vi "test - GB2312.vi"(8 "error in (no error)":errorcluster, 11 "TestCase in":refnum<class "labview-config-library.lvclass">) -> (0 "error out":errorcluster, 3 "TestCase out":refnum<class "labview-config-library.lvclass">)   [LabVIEW 2017, in "labview-config-library.lvclass"]
uses:
  labview-config-library.lvclass
  <vilib>/addons/_JKI Toolkits/VI Tester/TestCase.llb/TestCase.lvclass
  INI-Static-Variable-Support/LabVIEW-Config/LabVIEW-Config.lvclass
  INI-Static-Variable-Support/LabVIEW-Config/Read Key (String).vi
  C:/Program Files (x86)/National Instruments/LabVIEW 2017/vi.lib/addons/_JKI Toolkits/VI Tester/TestCase.llb/TestCase.lvclass
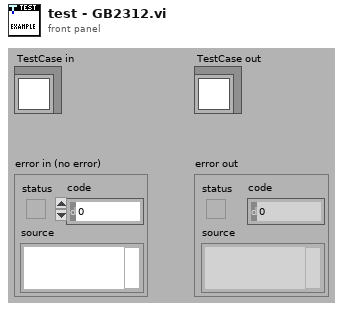
[diagram p1: front panel]
types:
  T1 = typedef "LabVIEW-Config.lvlib/LabVIEW-Config.lvclass/Config.ctl" = cluster{"Path":path, "Lines":string[], "Tokens":T2[], "Modified?":bool, "Cache":cluster{"Valid?":bool, "Key Information":T3[]}}
  T2 = typedef "LabVIEW-Config.lvlib/LabVIEW-Config.lvclass/LineToken.ctl" = enum8{"comment", "section", "key", "more"}
  T3 = typedef "LabVIEW-Config.lvlib/LabVIEW-Config.lvclass/KeyInfo.ctl" = cluster{"Key Indexes":cluster{"Indexes":i32[]}[], "Session Found?":bool, "Key found?":bool, "Session Index":i32}
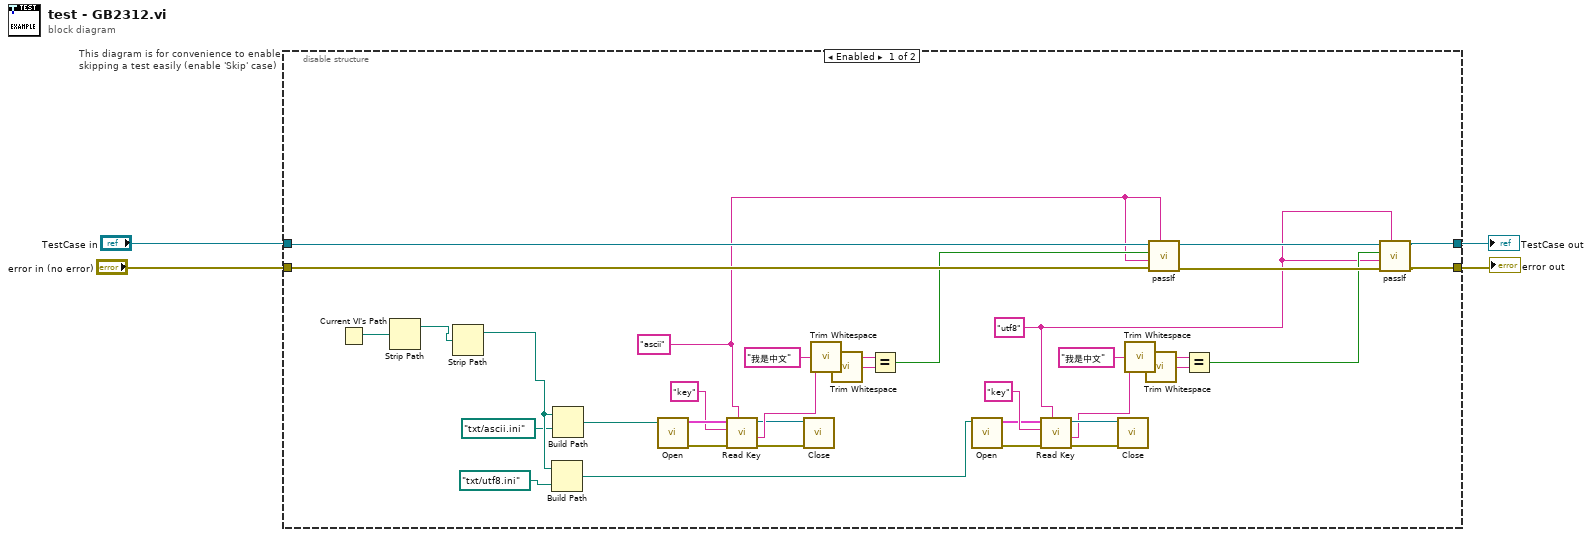
[diagram p0: block diagram]
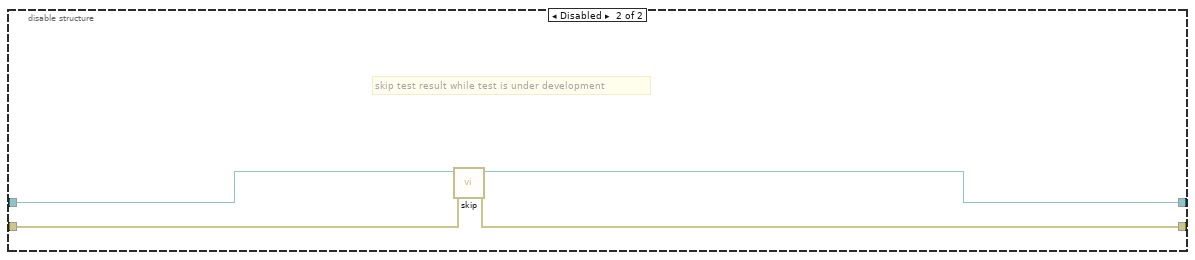
[diagram p2: hidden frame]
diagram:
  n1 = disable-structure "This diagram is for convenience to enable skipping a test easily (enable 'Skip' case)" shown="Enabled" {
    disable-tunnel: "TestCase in" -> [w12 w43]
    disable-tunnel: [w39 w41] -> w1
    disable-tunnel: [w38 w42] -> w3
    disable-tunnel: "error in (no error)" -> [w11 w40]
    frame Enabled {
      w5 = "utf8" ("Section Name")
      w7 = "ascii" ("Section Name")
      n2 = Current VI's Path() -> (path=w27:path)
      n3 = Strip Path(path=w27) -> (stripped path=w28:path)  [unwired: 1 out]
      n4 = Strip Path(path=w28) -> (stripped path=w29:path)  [unwired: 1 out]
      n5 = Build Path(base path=w29, name or relative path=path "txt/utf8.ini" ("file path (use dialog)")) -> (appended path=w13:path)
      n6 = Build Path(base path=w29, name or relative path=path "txt/ascii.ini" ("file path (use dialog)")) -> (appended path=w34:path)
      n7 = call "Open.vi"("Path"=w34) -> ("error out"=w31:errorcluster, "Config"=w30:T1)  [unwired: 7 in, 2 out]
      n8 = call-poly "Read Key.vi"("Section Name"=w7, "error in (no error)"=w31, "Key Name"="key", "Config in"=w30) -> ("error out"=w33:errorcluster, "Value"=w35:string, "Config out"=w32:refnum<class "LabVIEW-Config.lvclass">)  [unwired: 4 in, 1 out]
      n9 = call "Close.vi"("error in (no error)"=w33, "Config"=w32) -> ()  [unwired: 8 in, 2 out]
      n10 = call <vilib>:"Trim Whitespace.vi"("string"="我是中文" ("Section Name")) -> ("trimmed string"=w36:string)  [unwired: 1 in]
      n11 = call <vilib>:"Trim Whitespace.vi"("string"=w35) -> ("trimmed string"=w37:string)  [unwired: 1 in]
      n12 = Equal?(x=w36, y=w37) -> (x = y?=w10:bool)
      n13 = call "Open.vi"("Path"=w13) -> ("error out"=w19:errorcluster, "Config"=w20:T1)  [unwired: 7 in, 2 out]
      n14 = call-poly "Read Key.vi"("Section Name"=w5, "error in (no error)"=w19, "Key Name"="key", "Config in"=w20) -> ("error out"=w17:errorcluster, "Value"=w16:string, "Config out"=w18:refnum<class "LabVIEW-Config.lvclass">)  [unwired: 4 in, 1 out]
      n15 = call "Close.vi"("error in (no error)"=w17, "Config"=w18) -> ()  [unwired: 8 in, 2 out]
      n16 = call <vilib>:"Trim Whitespace.vi"("string"="我是中文" ("Section Name")) -> ("trimmed string"=w15:string)  [unwired: 1 in]
      n17 = call <vilib>:"Trim Whitespace.vi"("string"=w16) -> ("trimmed string"=w14:string)  [unwired: 1 in]
      n18 = call-dynamic "passIf.vi"("custom report message (\"\")"=w7, "error in (no error)"=w11, "message (\"\")"=w7, "pass"=w10, "TestCase in"=w12) -> ("error out"=w8:errorcluster, "TestCase out"=w9:refnum<class "labview-config-library.lvclass">)  [unwired: 5 in]
      n19 = Equal?(x=w15, y=w14) -> (x = y?=w6:bool)
      n20 = call-dynamic "passIf.vi"("custom report message (\"\")"=w5, "error in (no error)"=w8, "message (\"\")"=w5, "pass"=w6, "TestCase in"=w9) -> ("error out"=w38:errorcluster, "TestCase out"=w39:refnum<class "labview-config-library.lvclass">)  [unwired: 5 in]
    }
    frame Disabled {
      # "skip test result while test is under development"
      n21 = call <vilib>:"skip.vi"("error in (no error)"=w40, "TestCase in"=w43) -> ("error out"=w42:errorcluster, "TestCase out"=w41:refnum<class "labview-config-library.lvclass">)  [unwired: 8 in]
    }
  }
  "error out" <- w3
  "TestCase out" <- w1
